vi "Two_Counter.vi"() -> ()   [LabVIEW 2019]
uses:
  <vilib>/eio/EIONode/EIONode.xnode
  <vilib>/rvi/eio/common/nirviEmuTemplateMethod_errors.vi
panel:
  out "检测信号个数":u32
  out "时钟信号个数":u32
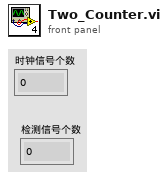
[diagram p1: front panel]
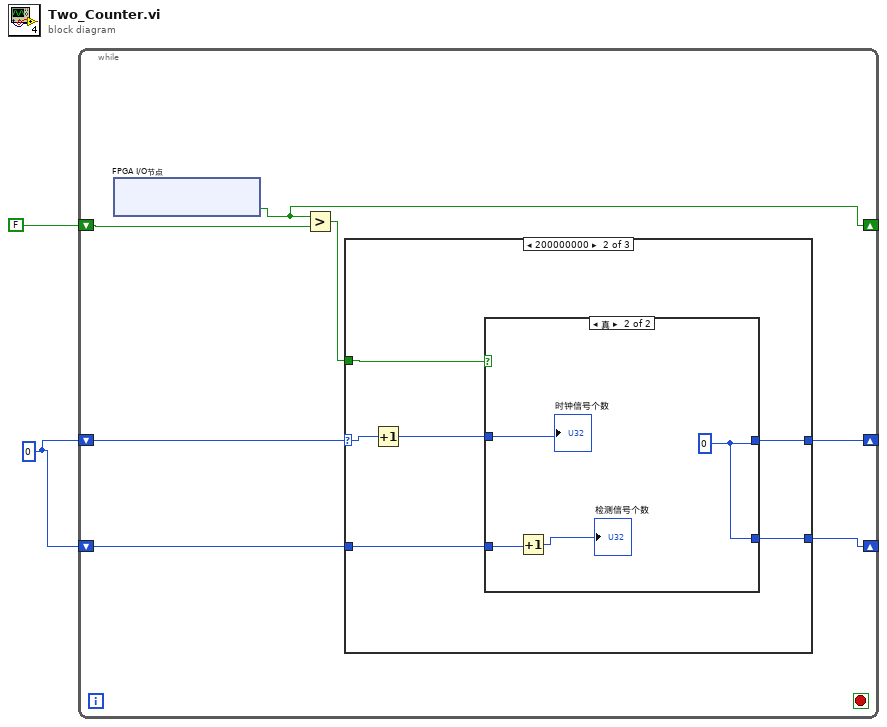
[diagram p0: block diagram]
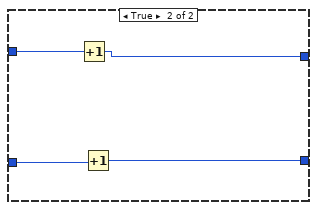
[diagram p3: hidden frame]
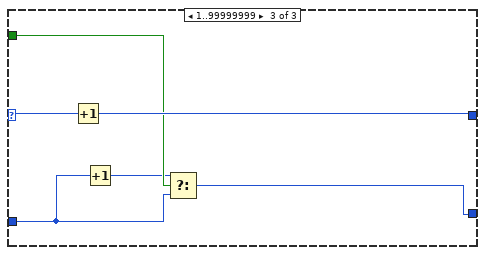
[diagram p5: hidden frame]
diagram:
  w1 = u32 0
  n1 = while {
    shift-right: [w8] -> _
    shift-left: FALSE -> [w9]
    shift-right: [w4] -> _
    shift-left: w1 -> [w7]
    shift-right: [w3] -> _
    shift-left: w1 -> [w5]
    stop <- _ stop-if-true
    n2 = xnode "FPGA I/O节点"() -> ("ConnectorB/DIO0"=w8:bool)  [unwired: 1 in, 1 out]
    n3 = Greater?(x=w8, y=w9) -> (0:w6:bool)
    n4 = case shown="200000000" w7 {
      selector: w7 -> [w13 w23 w34]
      tunnel: w6 -> [w14 w24 w32]
      tunnel: w5 -> [w10 w19 w31]
      tunnel: [w12 w21 w33] -> w4
      tunnel: [w11 w20 w29] -> w3
      frame 0, Default {
        n5 = case shown="假" w14 {
          tunnel: w13 -> [_ w18]
          tunnel: [_ w17] -> w12
          tunnel: w10 -> [_ w16]
          tunnel: [_ w15] -> w11
          frame False {
          }
          frame True {
            n6 = Increment(x=w18) -> (x+1=w17:u32)
            n7 = Increment(x=w16) -> (x+1=w15:u32)
          }
        }
      }
      frame 200000000 {
        n8 = Increment(x=w23) -> (x+1=w22:u32)
        n9 = case shown="真" w24 {
          tunnel: w22 -> [_ w26]
          tunnel: [_ w28] -> w21
          tunnel: [_ w28] -> w20
          tunnel: w19 -> [_ w27]
          frame False {
          }
          frame True {
            w28 = u32 0
            n10 = Increment(x=w27) -> (x+1=→"检测信号个数":u32)
            "时钟信号个数" <- w26
          }
        }
      }
      frame 1..99999999 {
        n11 = Increment(x=w34) -> (x+1=w33:u32)
        n12 = Increment(x=w31) -> (x+1=w30:u32)
        n13 = Select(t=w30, s=w32, f=w31) -> (s? t:f=w29:u32)
      }
    }
  }
